vi "WinCI Dialog - GetProjectNameAndPath.vi"(8 "error in (no error)":errorcluster, 9 "project path in":string, 10 "project name in":string) -> (0 "error out":errorcluster, 1 "project path out":string, 2 "project name out":string, 3 "cancelled?":bool)   [LabVIEW 2020, in "NI_SCC_WinCI.lvlib"]
uses:
  <vilib>/SourceControl/Providers/WinCI/NI_SCC_WinCI.lvlib
panel:
  in  "Source control project path":path
  in  "Source control project name":string
  in  "OK":bool
  in  "Cancel":bool
  in  "Help":bool
  # "The current source control provider does not support browsing to existing source control projects. Enter the project name and the path to the project."
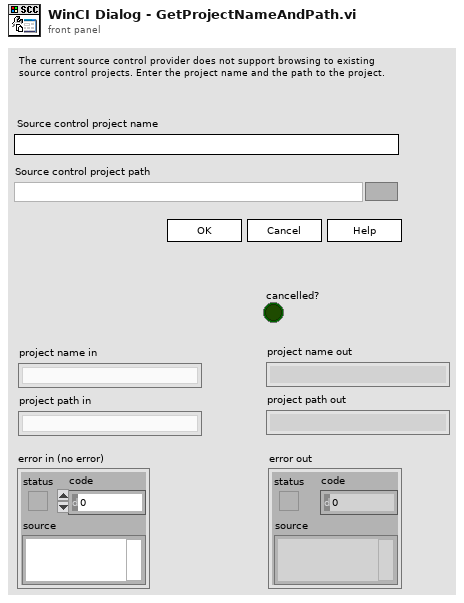
[diagram p1: front panel]
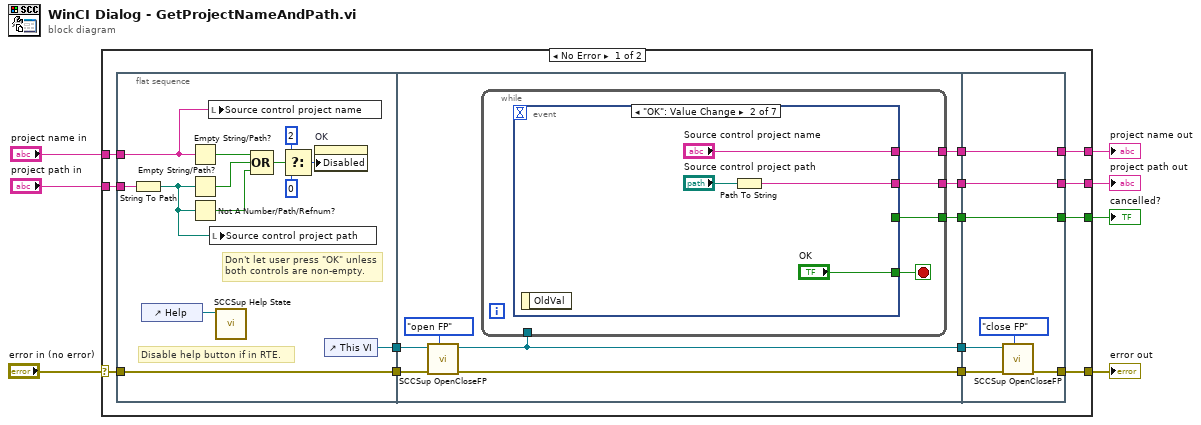
[diagram p0: block diagram]
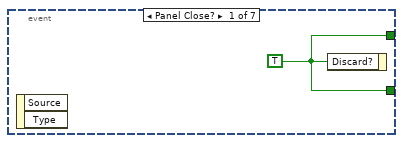
[diagram p2: hidden frame]
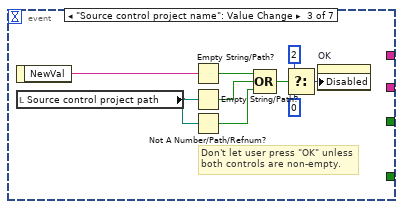
[diagram p3: hidden frame]
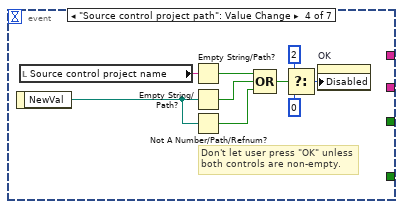
[diagram p4: hidden frame]
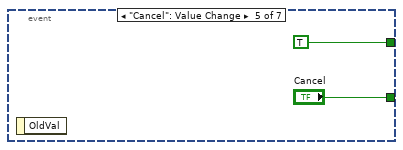
[diagram p5: hidden frame]
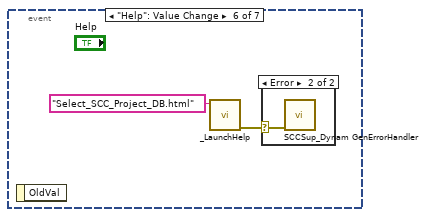
[diagram p6: hidden frame]
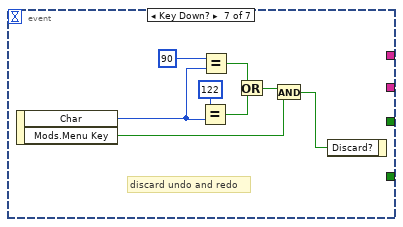
[diagram p8: hidden frame]
diagram:
  n1 = case shown="No Error" "error in (no error)" {
    selector: "error in (no error)" -> [w19 w90]
    tunnel: [w16 w90] -> w6
    tunnel: [w14 _] -> w5
    tunnel: "project name in" -> [w13 _]
    tunnel: "project path in" -> [w12 _]
    tunnel: [w9 _] -> w2
    tunnel: [w8 _] -> w1
    frame No Error {
      n2 = flat-sequence {
        tunnel: [w33] -> w21
        tunnel: w19 -> [w34]
        tunnel: [w34] -> w18
        tunnel: w13 -> [w31]
        tunnel: w12 -> [w32]
        tunnel: [w40] -> w20
        tunnel: w21 -> [w41]
        tunnel: w18 -> [w39]
        tunnel: [w38] -> w17
        tunnel: [w37] -> w15
        tunnel: [w36] -> w11
        tunnel: [w35] -> w10
        tunnel: w20 -> [w88]
        tunnel: w17 -> [w87]
        tunnel: [w86] -> w16
        tunnel: [w85] -> w14
        tunnel: w15 -> [w85]
        tunnel: w11 -> [w84]
        tunnel: w10 -> [w83]
        tunnel: [w84] -> w9
        tunnel: [w83] -> w8
        frame #0 {
          # "Disable help button if in RTE."
          # "Don't let user press \"OK\" unless both controls are non-empty."
          n3 = String To Path(string=w32) -> (path=w30:path)
          n4 = control-ref of="Help"() -> (w22:refnum<vi>)
          n5 = Empty String/Path?(string/path=w31) -> (empty?=w29:bool)
          n6 = Empty String/Path?(string/path=w30) -> (empty?=w28:bool)
          n7 = Not A Number/Path/Refnum?(number/path/refnum=w30) -> (NaN/Path/Refnum?=w27:bool)
          n8 = local write "Source control project name"(w31) -> ()
          n9 = local write "Source control project path"(w30) -> ()
          n10 = call <vilib>:"SCCSup Help State.vi"("help ref"=w22) -> ()  [unwired: 10 in, 1 out]
          n11 = Compound Arithmetic op=OR(w29, w28, w27) -> (w26:bool)
          n12 = Select(t=u8 2 ("Disabled"), s=w26, f=u8 0 ("Disabled")) -> (s? t:f=w24:u8)
          n13 = property on="OK" class="Bool"("Disabled"=w24) -> ()  [unwired: 2 in, 2 out]
          n14 = control-ref of="This VI"() -> (w33:refnum<vi>)
        }
        frame #1 {
          n15 = call <vilib>:"SCCSup OpenCloseFP.vi"("function"=enum16{"open FP", "close FP"}."open FP", "error in (no error)"=w39, "VI Refnum in"=w41) -> ("error out"=w38:errorcluster, "VI Refnum out"=w40:refnum<vi>)  [unwired: 7 in]
          n16 = while {
            tunnel: [w45] -> w37
            tunnel: w40 -> [_]
            tunnel: [w44] -> w36
            tunnel: [w43] -> w35
            stop <- w46 stop-if-true
            n17 = event shown="[1] \"OK\": Value Change" {
              selector: _ -> [_ _ _ _ _ _ _]
              dyn-events: _ -> [_ _ _ _ _ _ _]
              timeout: _ -> [_ _ _ _ _ _ _]
              tunnel: [w47 "OK" _ _ "Cancel" _ _] -> w46
              tunnel: [w47 _ _ _ TRUE _ _] -> w45
              tunnel: [_ "Source control project name" _ _ _ _ _] -> w43
              tunnel: [_ w48 _ _ _ _ _] -> w44
              event Panel Close? {
                w47 = TRUE
                n18 = event-data() -> ()  [unwired: 1 in, 2 out]
                n19 = event-data("Discard?"=w47) -> ()  [unwired: 1 in, 1 out]
              }
              event "OK": Value Change {
                n20 = event-data() -> ()  [unwired: 1 in, 1 out]
                n21 = Path To String(path="Source control project path") -> (string=w48:string)
              }
              event "Source control project name": Value Change {
                # "Don't let user press \"OK\" unless both controls are non-empty."
                n22 = event-data() -> ("NewVal"=w53:string)  [unwired: 1 in]
                n23 = local read "Source control project path"() -> (w52:path)
                n24 = Empty String/Path?(string/path=w53) -> (empty?=w54:bool)
                n25 = Empty String/Path?(string/path=w52) -> (empty?=w55:bool)
                n26 = Not A Number/Path/Refnum?(number/path/refnum=w52) -> (NaN/Path/Refnum?=w56:bool)
                n27 = Compound Arithmetic op=OR(w54, w55, w56) -> (w57:bool)
                n28 = Select(t=u8 2 ("Disabled"), s=w57, f=u8 0 ("Disabled")) -> (s? t:f=w59:u8)
                n29 = property on="OK" class="Bool"("Disabled"=w59) -> ()  [unwired: 2 in, 2 out]
              }
              event "Source control project path": Value Change {
                # "Don't let user press \"OK\" unless both controls are non-empty."
                n30 = event-data() -> ("NewVal"=w62:path)  [unwired: 1 in]
                n31 = local read "Source control project name"() -> (w61:string)
                n32 = Empty String/Path?(string/path=w61) -> (empty?=w63:bool)
                n33 = Empty String/Path?(string/path=w62) -> (empty?=w64:bool)
                n34 = Not A Number/Path/Refnum?(number/path/refnum=w62) -> (NaN/Path/Refnum?=w65:bool)
                n35 = Compound Arithmetic op=OR(w63, w64, w65) -> (w66:bool)
                n36 = Select(t=u8 2 ("Disabled"), s=w66, f=u8 0 ("Disabled")) -> (s? t:f=w68:u8)
                n37 = property on="OK" class="Bool"("Disabled"=w68) -> ()  [unwired: 2 in, 2 out]
              }
              event "Cancel": Value Change {
                n38 = event-data() -> ()  [unwired: 1 in, 1 out]
              }
              event "Help": Value Change {
                n39 = event-data() -> ()  [unwired: 1 in, 1 out]
                n40 = call <helpdir>:"_LaunchHelp.vi"("HTML filename"="Select_SCC_Project_DB.html" ("Help topic")) -> ("error out"=w73:errorcluster)  [unwired: 6 in]
                n41 = case shown="Error" w73 {
                  selector: w73 -> [_ w74]
                  frame No Error {
                  }
                  frame Error {
                    n42 = call <vilib>:"SCCSup_Dynam GenErrorHandler.vi"("error in (no error)"=w74) -> ()  [unwired: 9 in, 2 out]
                  }
                }
              }
              event Key Down? {
                # "discard undo and redo"
                n43 = event-data() -> ("Char"=w77:i16, "Mods.Menu Key"=w76:bool)  [unwired: 1 in]
                n44 = Equal?(x=i16 122, y=w77) -> (x = y?=w80:bool)
                n45 = Equal?(x=i16 90, y=w77) -> (x = y?=w79:bool)
                n46 = Or(x=w79, y=w80) -> (x .or. y?=w78:bool)
                n47 = And(x=w78, y=w76) -> (x .and. y?=w75:bool)
                n48 = event-data("Discard?"=w75) -> ()  [unwired: 1 in, 1 out]
              }
            }
          }
        }
        frame #2 {
          n49 = call <vilib>:"SCCSup OpenCloseFP.vi"("function"=enum16{"open FP", "close FP"}."close FP", "error in (no error)"=w87, "VI Refnum in"=w88) -> ("error out"=w86:errorcluster)  [unwired: 7 in, 1 out]
        }
      }
    }
    frame Error {
    }
  }
  "error out" <- w6
  "cancelled?" <- w5
  "project name out" <- w1
  "project path out" <- w2
